vi "GUI_HamamatsuSpectrometer_v2.0.0.vi"() -> ()   [LabVIEW 2013]
uses:
  Shared/GUI_Template/GUI_master/tcp_new_data_event.ctl
  Shared/GUI_Template/GUI_master/tcp new data cluster.ctl
  <vilib>/Utility/miscctls.llb/LVOffsetAndMultiplierTypeDef.ctl
panel:
  out "wavelength::1":dbl[](array[numeric]) caption="wavelength"
  in  "Local Saving Path":path
  in  "stop":bool
  out "FWHM::1":dbl caption="FWHM" min=0.0 max=10000.0
  in  "BGlevel::1":dbl caption="BGlevel" min=0.0 max=10000.0
  out "MeanWavelength::1":dbl caption="MeanWavelength" min=0.0 max=10000.0
  out "lambda_r::1":dbl caption="lambda_r" min=0.0 max=10000.0
  out "lambda_b::1":dbl caption="lambda_b" min=0.0 max=10000.0
  out "lambda_width (SD)::1":dbl caption="lambda_width (SD)" min=0.0 max=10000.0
  out "AverageCountLevel::1":dbl caption="AverageCountLevel" min=0.0 max=10000.0
  in  "exposure::1":dbl caption="exposure" min=1.0 max=300.0
  in  "trigger::1":bool caption="trigger"
  in  "save::1":bool caption="save"
  in  "shotnumber":i32
  in  "Refresh Button":bool
  in  "GUIdevice 1":string="P2-AndorCam"
  out "counts::1":dbl[](array[numeric]) caption="counts"
  out "tcp data event":T1
  out "UDP error message":string caption="Device Errors"
  out "XY Graph":cluster{"Value":dbl[], "Value":dbl[]}[](graph)
  out "Intensity Graph":dbl[][](graph)
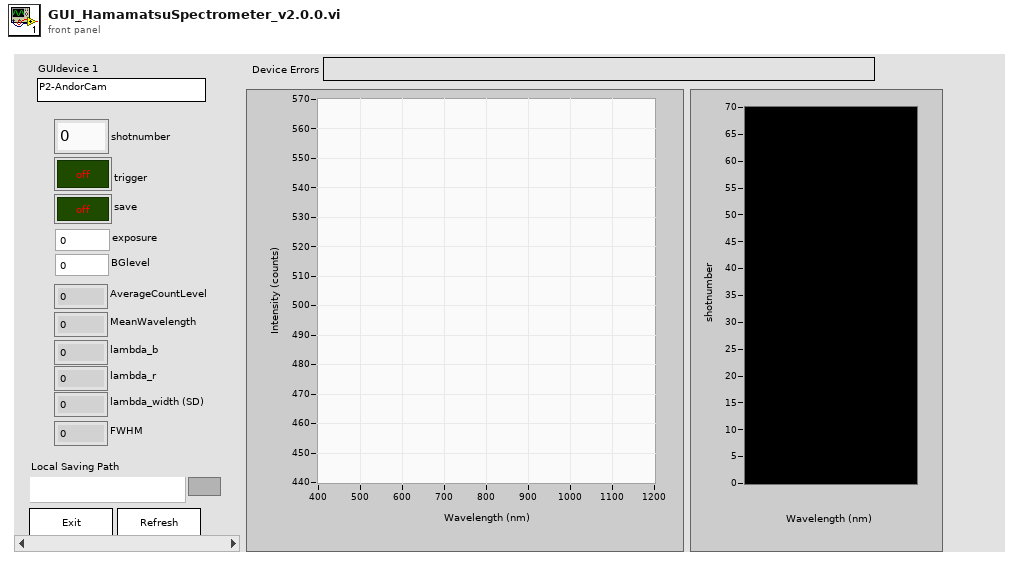
[diagram p1: front panel]
types:
  T1 = typedef "tcp_new_data_event.ctl" = refnum<user-event>
  T2 = enum32{"invalid app kind", "Development System", "Run Time System", "Student Edition", "Embedded LabVIEW", "Evaluation", "Custom"}
  T3 = typedef "tcp new data cluster.ctl" = cluster{"EventEnum":enum16{"new data", "connection status update"}, "Device name":string}
  T4 = enum32{"Invalid", "Standard", "Closed", "Hidden", "Minimized", "Maximized"}
  T5 = typedef "LVOffsetAndMultiplierTypeDef.ctl" = cluster{"Offset":dbl, "Multiplier":dbl}
  T6 = cluster{"Core":cluster{"Current VI Reference":refnum<vi>, "Close Panel on Exit?":bool}, "Your Boolean data":bool, "Your string data":string, "SuperGUI":cluster{"STOP queue":refnum<queue>, "SuperGUI ref":refnum<vi>}, "Graph":cluster{"XY Graph":cluster{"Value":dbl[], "Value":dbl[]}, "Intensity Graph":dbl[][], "Shot Number":i32}}
  T7 = cluster{"XY Graph":cluster{"Value":dbl[], "Value":dbl[]}, "Intensity Graph":dbl[][], "Shot Number":i32}
  T8 = cluster{"STOP queue":refnum<queue>, "SuperGUI ref":refnum<vi>}
  T9 = cluster{"Current VI Reference":refnum<vi>, "Close Panel on Exit?":bool}
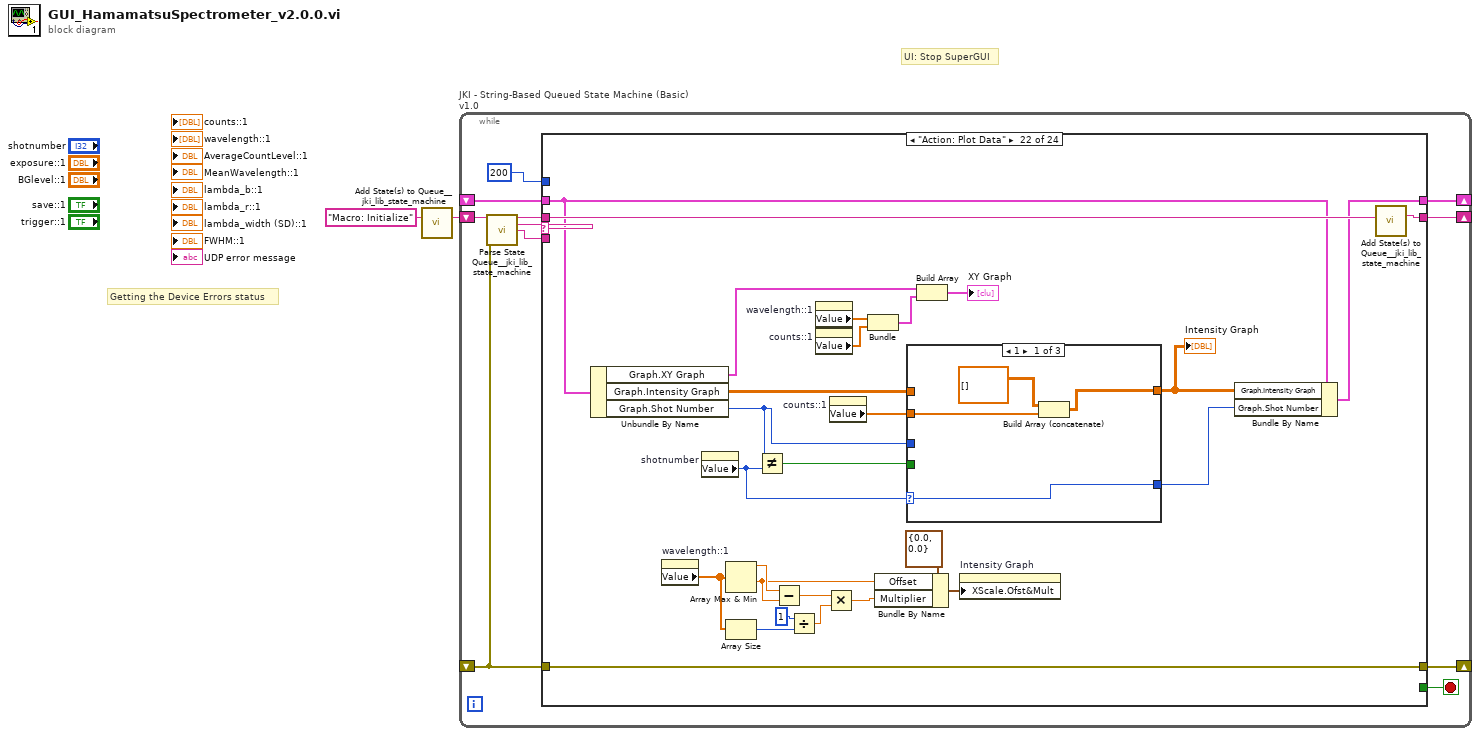
[diagram p0: block diagram]
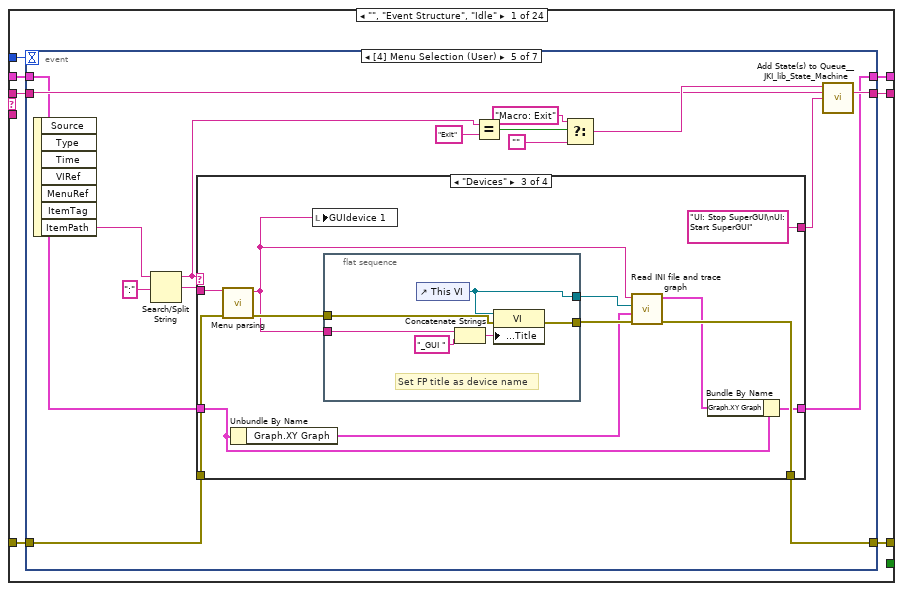
[diagram p2: hidden frame]
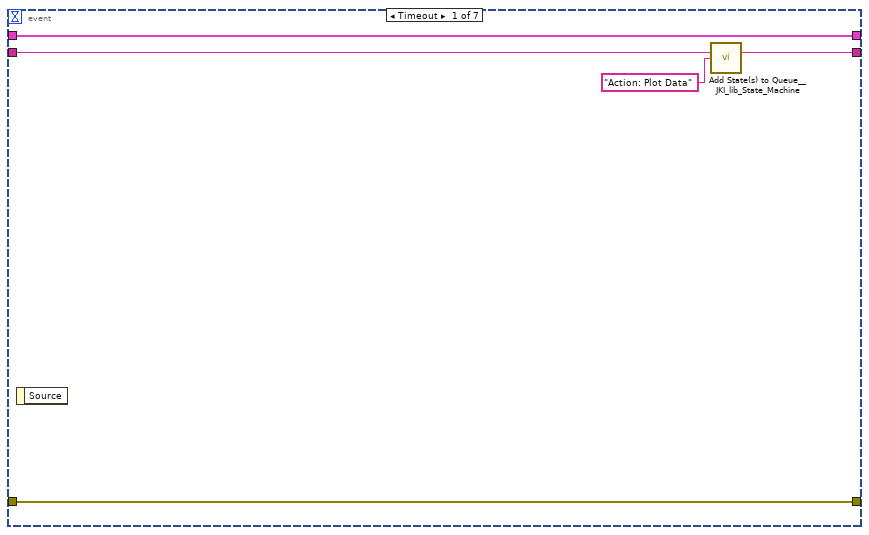
[diagram p3: hidden frame]
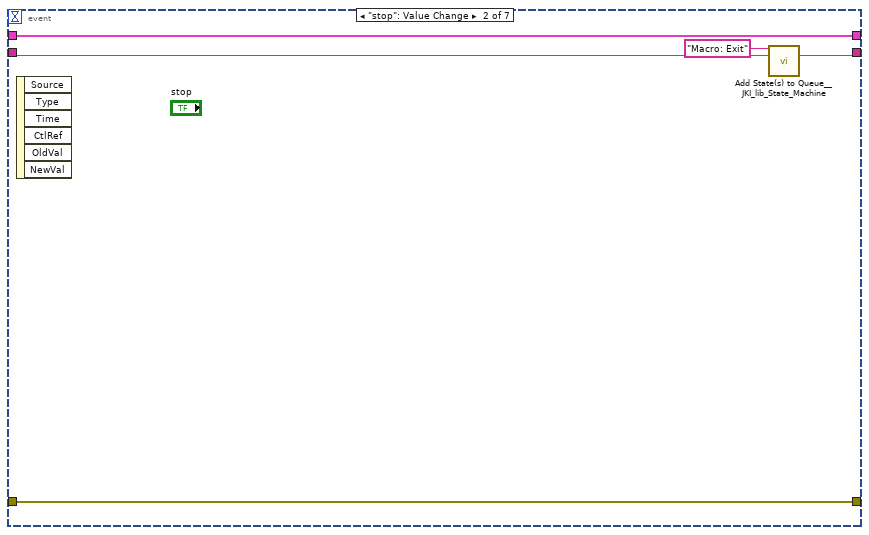
[diagram p4: hidden frame]
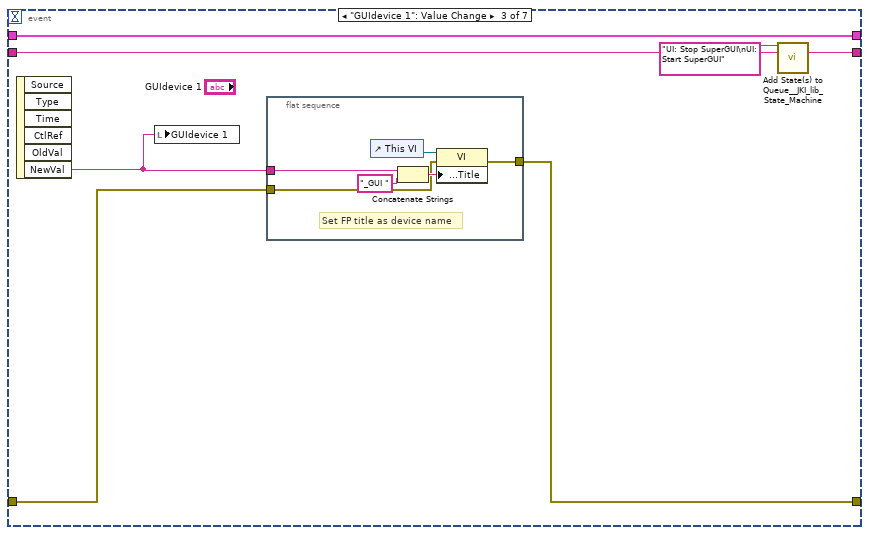
[diagram p5: hidden frame]
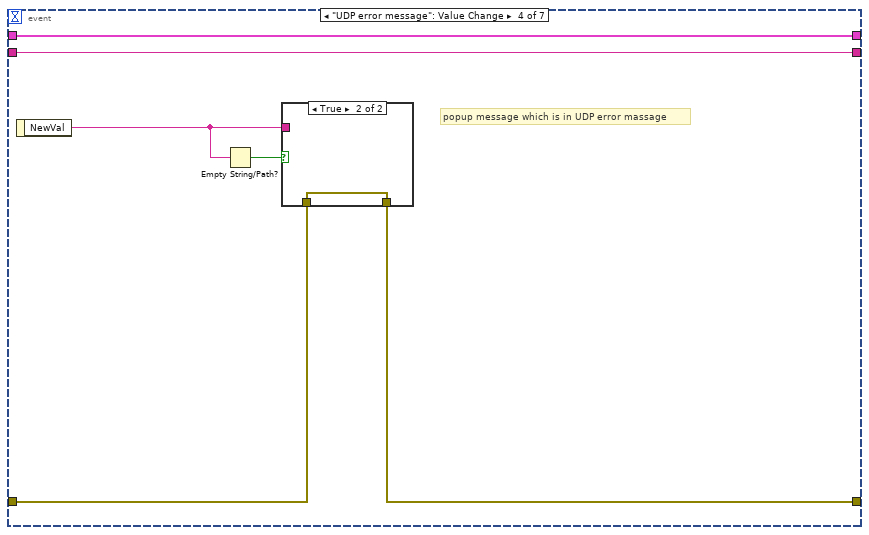
[diagram p6: hidden frame]
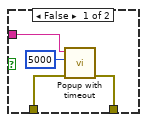
[diagram p7: hidden frame]
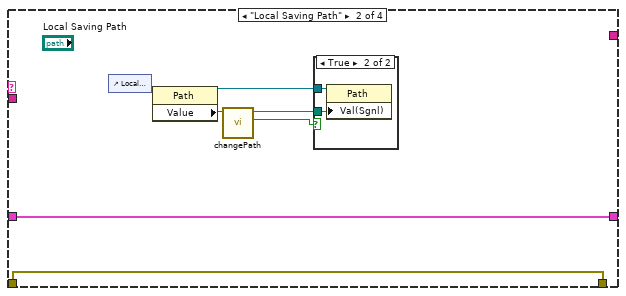
[diagram p9: hidden frame]
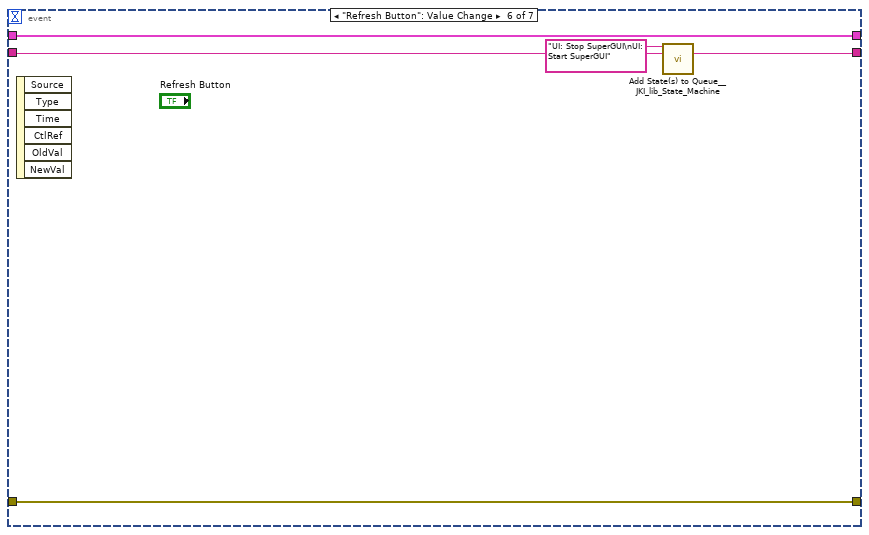
[diagram p12: hidden frame]
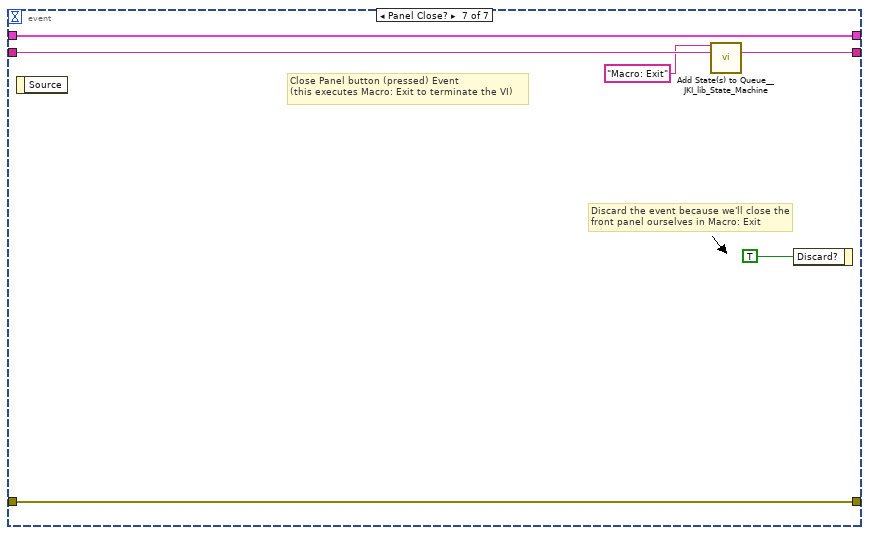
[diagram p13: hidden frame]
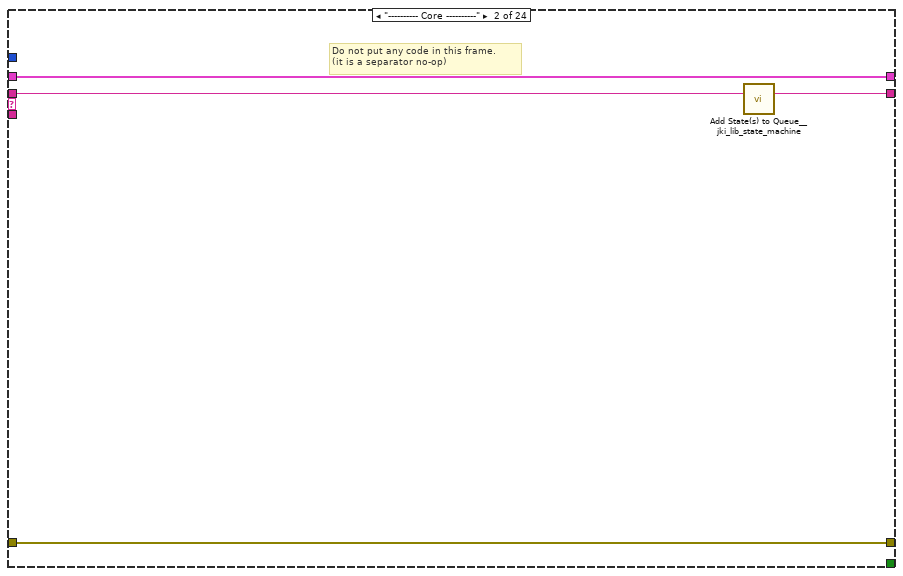
[diagram p14: hidden frame]
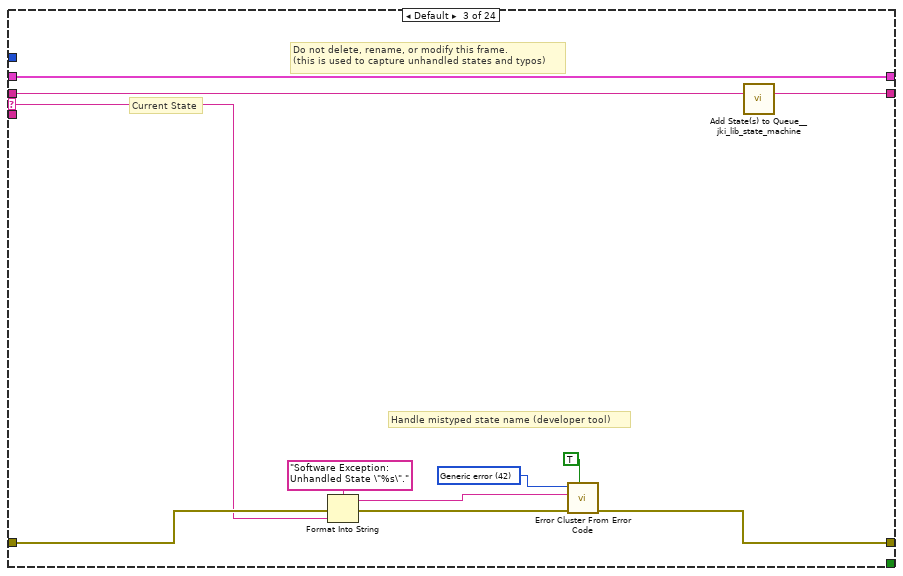
[diagram p15: hidden frame]
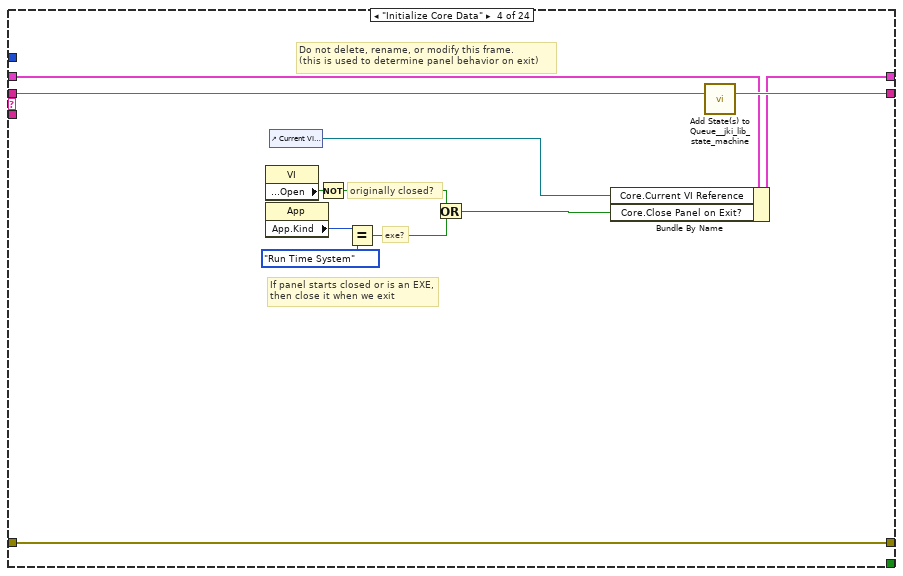
[diagram p16: hidden frame]
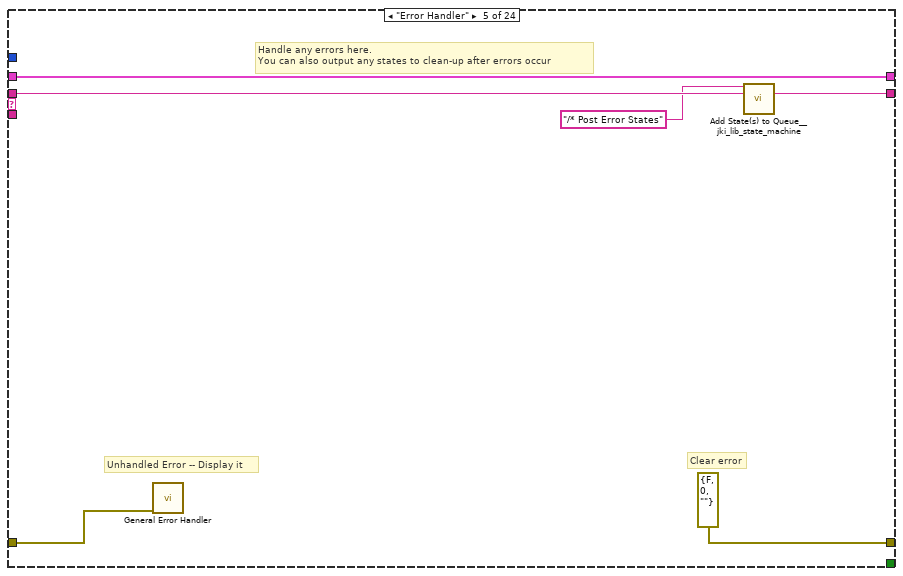
[diagram p17: hidden frame]
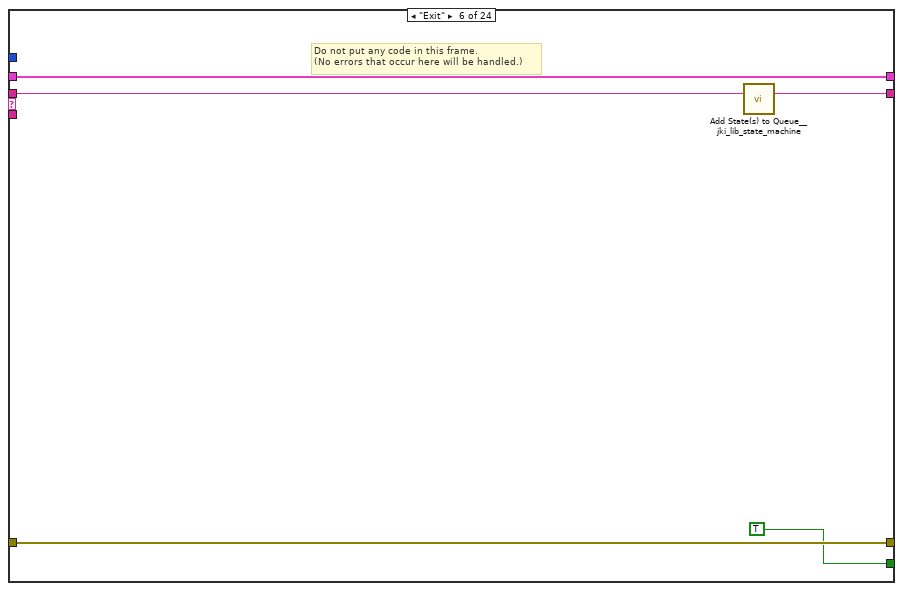
[diagram p18: hidden frame]
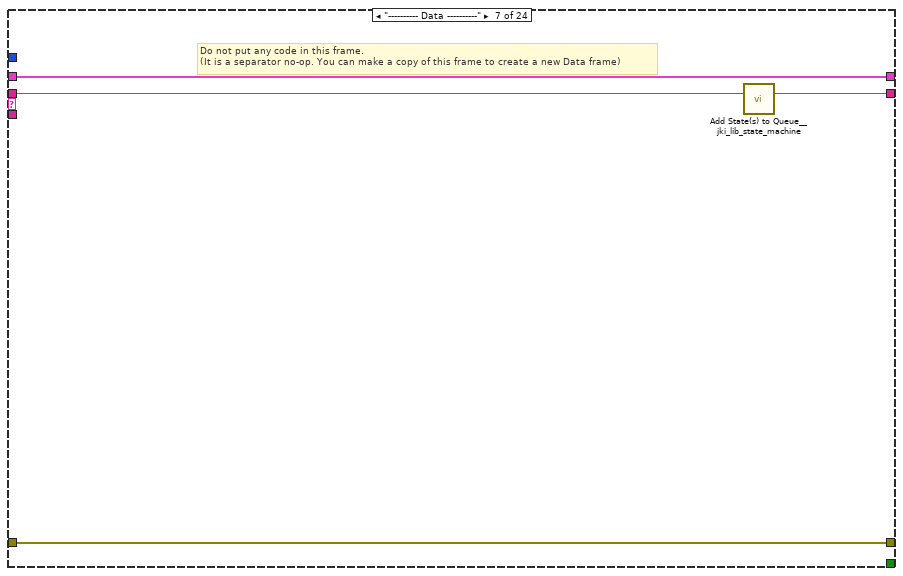
[diagram p19: hidden frame]
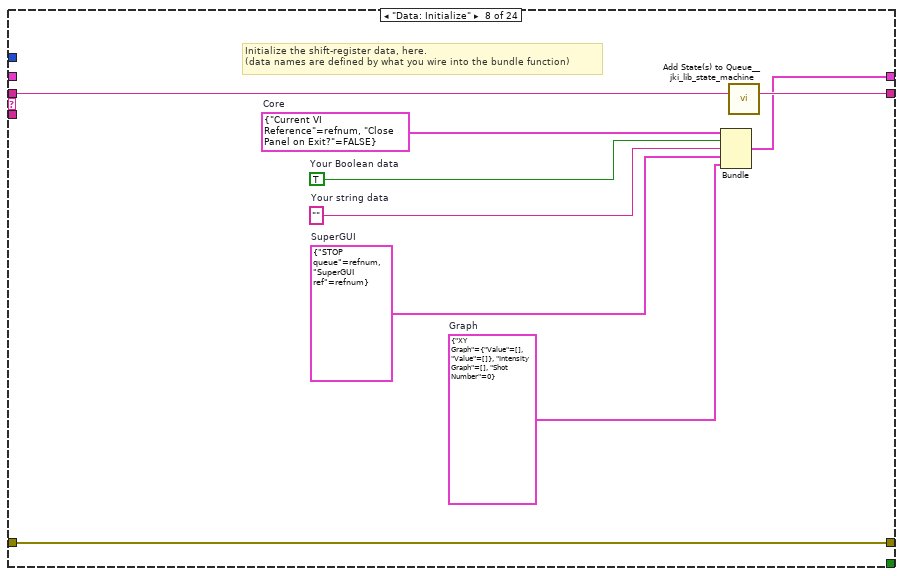
[diagram p20: hidden frame]
diagram:
  # "UI: Stop SuperGUI"
  # "Getting the Device Errors status"
  n1 = call <vilib>:"Add State(s) to Queue__jki_lib_state_machine.vi"("State(s) in (\"\")"="Macro: Initialize") -> ("States Out"=w2:string)  [unwired: 14 in]
  n2 = while "JKI - String-Based Queued State Machine (Basic) v1.0" {
    shift-right: [w6] -> _
    shift-left: _ -> [w5]
    shift-right: [w9] -> _
    shift-left: _ -> [w3]
    shift-right: [w8] -> _
    shift-left: w2 -> [w10]
    stop <- w7 stop-if-true
    n3 = call <vilib>:"Parse State Queue__jki_lib_state_machine.vi"("State Queue"=w10, "Error In (no error)"=w3) -> ("Remaining States"=w12:string, "Current State"=w13:string, "Arguments"=w11:string)  [unwired: 11 in]
    n4 = case shown="\"Action: Plot Data\"" w13 {
      selector: w13 -> [_ _ w116 _ _ _ _ _ _ _ _ _ _ _ _ _ _ _ _ _ _ _ _ _]
      tunnel: w12 -> [w20 w115 w120 w138 w144 w149 w153 w162 w168 w172 w176 w185 w221 w255 w263 w269 w280 w306 w311 w322 w326 w353 w376 w386]
      tunnel: w11 -> [_ _ _ _ _ _ _ _ _ _ _ _ _ _ _ w264 w274 _ _ _ _ _ _ _]
      tunnel: w5 -> [w18 w112 w118 w129 w141 w147 w150 _ w163 w169 w174 w183 w219 w246 w258 w267 w276 w303 w308 w319 w323 w345 w373 w380]
      tunnel: [w17 w113 w122 w135 errorcluster {"status"=FALSE, "code"=0, "source"=""} ("error out") w146 w151 w159 w164 w170 w173 w181 w216 w239 w256 w265 w277 w304 w309 w320 w324 w351 w374 w381] -> w9
      tunnel: w3 -> [w16 w113 w121 w135 w140 w146 w151 w159 w165 w170 w173 w182 w217 w240 w257 w266 w278 w304 w309 w320 w324 w351 w374 w382]
      tunnel: [w19 w114 w119 w137 w143 w148 w152 w161 w167 w171 w175 w184 w220 w254 w262 w268 w279 w305 w310 w321 w325 w352 w375 w385] -> w8
      tunnel: [_ _ _ _ _ TRUE _ _ _ _ _ _ _ _ _ _ _ _ _ _ _ _ _ _] -> w7
      tunnel: [w15 w112 w118 w136 w141 w147 w150 w160 w163 w169 w174 w183 w219 w245 w258 w267 w276 w303 w308 w319 w323 w344 w373 w379] -> w6
      tunnel: 200 ("time to wait (main loop)") -> [w14 _ _ _ _ _ _ _ _ _ _ _ _ _ _ _ _ _ _ _ _ _ _ _]
      frame "", "Event Structure", "Idle" {
        n5 = event shown="[4] Menu Selection (User)" {
          selector: _ -> [_ _ _ _ _ _ _]
          dyn-events: _ -> [_ _ _ _ _ _ _]
          timeout: w14 -> [_ _ _ _ _ _ _]
          tunnel: w20 -> [w25 w28 w34 w48 w65 w103 w111]
          tunnel: [w24 w27 w33 w48 w64 w102 w110] -> w19
          tunnel: w18 -> [w21 w30 w37 w49 w56 w105 w108]
          tunnel: [w22 w29 w35 w44 w58 w104 w109] -> w17
          tunnel: w16 -> [w22 w29 w36 w45 w59 w104 w109]
          tunnel: [w21 w30 w37 w49 w55 w105 w108] -> w15
          event Timeout {
            n6 = event-data() -> ()  [unwired: 1 in, 1 out]
            n7 = call <vilib>:"Add State(s) to Queue__JKI_lib_State_Machine.vi"("State(s) in (\"\")"=w25, "State(s) at Back (\"\")"="Action: Plot Data" ("State(s) in Front (\"\")")) -> ("States Out"=w24:string)  [unwired: 13 in]
          }
          event "stop": Value Change {
            n8 = event-data() -> ()  [unwired: 1 in, 6 out]
            n9 = call <vilib>:"Add State(s) to Queue__JKI_lib_State_Machine.vi"("State(s) in Front (\"\")"="Macro: Exit", "State(s) in (\"\")"=w28) -> ("States Out"=w27:string)  [unwired: 13 in]
          }
          event "GUIdevice 1": Value Change {
            n10 = event-data() -> ("NewVal"=w31:string)  [unwired: 1 in, 5 out]
            n11 = local write "GUIdevice 1"(w31) -> ()
            n12 = flat-sequence {
              tunnel: [w40] -> w35
              tunnel: w36 -> [w39]
              tunnel: w31 -> [w38]
              frame #0 {
                # "Set FP title as device name"
                n13 = control-ref of="This VI"() -> (w43:refnum<vi>)
                n14 = Concatenate Strings(w38, "_GUI ") -> (w42:string)
                n15 = property class="VI"(reference=w43, error in=w39, "Front Panel.Title"=w42) -> (error out=w40:errorcluster)  [unwired: 1 out]
              }
            }
            n16 = call <vilib>:"Add State(s) to Queue__JKI_lib_State_Machine.vi"("State(s) in Front (\"\")"="UI: Stop SuperGUI\nUI: Start SuperGUI", "State(s) in (\"\")"=w34) -> ("States Out"=w33:string)  [unwired: 13 in]
          }
          event "UDP error message": Value Change {
            # "popup message which is in UDP error massage"
            n17 = event-data() -> ("NewVal"=w46:string)  [unwired: 1 in]
            n18 = Empty String/Path?(string/path=w46) -> (empty?=w47:bool)
            n19 = case shown="True" w47 {
              tunnel: w46 -> [w53 _]
              tunnel: w45 -> [w52 w54]
              tunnel: [w51 w54] -> w44
              frame False {
                n20 = call "Popup with timeout.vi"("error"=w52, "timeout"=u32 5000, "message"=w53) -> ("error out"=w51:errorcluster)  [unwired: 8 in]
              }
              frame True {
              }
            }
          }
          event Menu Selection (User) {
            n21 = event-data() -> ("ItemPath"=w61:string)  [unwired: 1 in, 6 out]
            n22 = Search/Split String(string=w61, search string/char (-)=":") -> (substring before match=w57:string, match + rest of string=w60:string)  [unwired: 1 in, 1 out]
            n23 = case shown="\"Devices\"" w57 {
              tunnel: w60 -> [_ _ w92 _]
              tunnel: w59 -> [w72 w79 w91 w100]
              tunnel: [w72 w79 w86 w100] -> w58
              tunnel: [_ _ "UI: Stop SuperGUI\nUI: Start SuperGUI" _] -> w63
              tunnel: w56 -> [w71 w78 w84 w99]
              tunnel: [w71 w78 w82 w99] -> w55
              frame "", Default {
              }
              frame "Local Saving Path" {
                n24 = control-ref of="Local Saving Path"() -> (w77:refnum<vi>)
                n25 = property class="Path"(reference=w77) -> (reference out=w74:refnum<vi>, "Value"=w73:path)  [unwired: 1 in, 1 out]
                n26 = call "changePath.vi"("Local Saving in (h)"=w73) -> ("change (h)"=w75:bool, "Local Saving out (h)"=w76:path)  [unwired: 9 in]
                n27 = case shown="True" w75 {
                  tunnel: w74 -> [_ w81]
                  tunnel: w76 -> [_ w80]
                  frame False {
                  }
                  frame True {
                    n28 = property class="Path"(reference=w81, "Val(Sgnl)"=w80) -> ()  [unwired: 1 in, 2 out]
                  }
                }
              }
              frame "Devices" {
                n29 = call "Menu parsing.vi"("ItemPath 3"=w92) -> ("ItemPath 2"=w89:string)  [unwired: 9 in, 1 out]
                n30 = Unbundle By Name(w84) -> ("Graph.XY Graph"=w85:cluster{"Value":dbl[], "Value":dbl[]})
                n31 = local write "GUIdevice 1"(w89) -> ()
                n32 = flat-sequence {
                  tunnel: [w96] -> w87
                  tunnel: w91 -> [w95]
                  tunnel: w89 -> [w94]
                  tunnel: [w93] -> w88
                  frame #0 {
                    # "Set FP title as device name"
                    n33 = control-ref of="This VI"() -> (w93:refnum<vi>)
                    n34 = Concatenate Strings(w94, "_GUI ") -> (w98:string)
                    n35 = property class="VI"(reference=w93, error in=w95, "Front Panel.Title"=w98) -> (error out=w96:errorcluster)  [unwired: 1 out]
                  }
                }
                n36 = call "Read INI file and trace graph.vi"("error in (no error)"=w87, "XY Graph in"=w85, "This VI"=w88, "Device Name"=w89) -> ("error out"=w86:errorcluster, "XY Graph out"=w83:cluster{"Value":dbl[], "Value":dbl[]})  [unwired: 6 in]
                n37 = Bundle By Name(cluster=w84, "Graph.XY Graph"=w83) -> (w82:T6)
              }
              frame "Exit" {
              }
            }
            n38 = Equal?(x=w57, y="Exit") -> (x = y?=w69:bool)
            n39 = Select(t="Macro: Exit", s=w69, f="") -> (s? t:f=w66:string)
            n40 = call <vilib>:"Add State(s) to Queue__JKI_lib_State_Machine.vi"("State(s) in Front (\"\")"=w66, "State(s) in (\"\")"=w65, "State(s) at Back (\"\")"=w63) -> ("States Out"=w64:string)  [unwired: 12 in]
          }
          event "Refresh Button": Value Change {
            n41 = event-data() -> ()  [unwired: 1 in, 6 out]
            n42 = call <vilib>:"Add State(s) to Queue__JKI_lib_State_Machine.vi"("State(s) in Front (\"\")"="UI: Stop SuperGUI\nUI: Start SuperGUI", "State(s) in (\"\")"=w103) -> ("States Out"=w102:string)  [unwired: 13 in]
          }
          event Panel Close? {
            # "Discard the event because we'll close the front panel ourselves in Macro: Exit"
            # "Close Panel button (pressed) Event\n(this executes Macro: Exit to terminate the VI)"
            n43 = event-data() -> ()  [unwired: 1 in, 1 out]
            n44 = call <vilib>:"Add State(s) to Queue__JKI_lib_State_Machine.vi"("State(s) in Front (\"\")"="Macro: Exit", "State(s) in (\"\")"=w111) -> ("States Out"=w110:string)  [unwired: 13 in]
            n45 = event-data("Discard?"=TRUE) -> ()  [unwired: 1 in, 1 out]
          }
        }
      }
      frame "---------- Core ----------" {
        # "Do not put any code in this frame.\n(it is a separator no-op)"
        n46 = call <vilib>:"Add State(s) to Queue__jki_lib_state_machine.vi"("State(s) in (\"\")"=w115) -> ("States Out"=w114:string)  [unwired: 14 in]
      }
      frame Default {
        w125 = 42 items=["No error", "Argument error", "Memory is full", "Out of zone", "End of file", "File already open", "Generic file I/O error", "File not found", "File permission error", "Disk is full", "Duplicate path", "Too many files open", "System feature not enabled", "Resource file not found", "Cannot add resource", "Resource not found", "Image not found", "Image memory error", "Pen does not exist", "Config type invalid", "Config token not found", "Config parse error", "Config memory error", "Bad external code format", "Bad external code offset", "External code not present", "Null window", "Destroy window error", "Null menu", "Print aborted", "Bad print record", "Print driver error", "Windows error during printing", "Memory error during printing", "Print dialog error", "Generic print error", "Invalid device refnum", "Device not found", "Device parameter error", "Device unit error", "Cannot open device", "Device call aborted", "Generic error", "Cancelled by user", "Object ID too low", "Object ID too high", "Object not in heap", "Unknown heap", "Unknown object (invalid DefProc)", "Unknown object (DefProc not in table)", "Message out of range", "Invalid (null) method", "Unknown message", "Manager call not supported", "Bad address", "Network operation in progress", "Network operation timed out", "Connection is busy", "Network attribute not supported", "Network error", "Address in use", "System out of memory", "Connection aborted", "Connection refused", "Not connected", "Already connected", "Connection closed", "Initialization error (interapplication manager)", "Bad occurrence", "Wait on unbound occurrence handler", "Occurrence queue overflow", "Datalog type conflict", "Unused", "Unrecognized type (interapplication manager)", "Memory corrupt", "Failed to make temporary DLL", "Old CIN version", "Drag socket not found", "Failed to load drop-object", "Failed to register OLE object", "Failed to release OLE object", "Format specifier type mismatch", "Unknown format specifier", "Too few format specifiers", "Too many format specifiers", "Scan failed", "Newer CIN version", "Error converting to variant", "Runtime menu error", "Password tampered", "Variant attribute not found", "Incompatible variant data type", "Event data is not available", "Event Store is not present", "Occurrence is not found", "Event Queue is not created", "Event info is not available", "Refnum passed is NULL", "Error retrieving Class GUID", "Error retrieving CoClass GUID", "Error retrieving TypeLib GUID.", "Bad built application magic bytes.", "Specific driver is different from the specific driver associated with the Logical Name.", "There is no session opened to the class driver.", "Max Error", "MAX - Error with config objects", "MAX - Error loading configuration", "MAX - Group not supported"]
        # "Current State"
        # "Do not delete, rename, or modify this frame.\n(this is used to capture unhandled states and typos)"
        # "Handle mistyped state name (developer tool)"
        n47 = Format Into String(format string="Software Exception: Unhandled State \"%s\"." ("message"), error in=w121, w116) -> (resulting string=w124:string, error out=w123:errorcluster)  [unwired: 1 in]
        n48 = call <vilib>:"Error Cluster From Error Code.vi"("show call chain? (False)"=TRUE, "error in (no error)"=w123, "error message (\"\")"=w124, "error code (0)"=w125) -> ("error out"=w122:errorcluster)  [unwired: 5 in]
        n49 = call <vilib>:"Add State(s) to Queue__jki_lib_state_machine.vi"("State(s) in (\"\")"=w120) -> ("States Out"=w119:string)  [unwired: 14 in]
      }
      frame "Initialize Core Data" {
        # "Do not delete, rename, or modify this frame.\n(this is used to determine panel behavior on exit)"
        # "originally closed?"
        # "exe?"
        # "If panel starts closed or is an EXE, then close it when we exit"
        n50 = property class="VI"() -> ("Front Panel.Open"=w134:bool)  [unwired: 2 in, 2 out]
        n51 = property class="App"() -> ("App.Kind"=w133:T2)  [unwired: 2 in, 2 out]
        n52 = control-ref of="Current VI Reference"() -> (w127:refnum<vi>)
        n53 = Not(x=w134) -> (.not. x?=w131:bool)
        n54 = Equal?(x=w133, y=T2."Run Time System" ("Application:Kind")) -> (x = y?=w130:bool)
        n55 = Or(x=w131, y=w130) -> (x .or. y?=w128:bool)
        n56 = Bundle By Name(cluster=w129, "Core.Current VI Reference"=w127, "Core.Close Panel on Exit?"=w128) -> (w136:T6)
        n57 = call <vilib>:"Add State(s) to Queue__jki_lib_state_machine.vi"("State(s) in (\"\")"=w138) -> ("States Out"=w137:string)  [unwired: 14 in]
      }
      frame "Error Handler" {
        # "Unhandled Error -- Display it"
        # "Handle any errors here.\nYou can also output any states to clean-up after errors occur"
        # "Clear error"
        n58 = call <vilib>:"General Error Handler.vi"("error in (no error)"=w140) -> ()  [unwired: 10 in, 5 out]
        n59 = call <vilib>:"Add State(s) to Queue__jki_lib_state_machine.vi"("State(s) in Front (\"\")"="/* Post Error States", "State(s) in (\"\")"=w144) -> ("States Out"=w143:string)  [unwired: 13 in]
      }
      frame "Exit" {
        # "Do not put any code in this frame.\n(No errors that occur here will be handled.)"
        n60 = call <vilib>:"Add State(s) to Queue__jki_lib_state_machine.vi"("State(s) in (\"\")"=w149) -> ("States Out"=w148:string)  [unwired: 14 in]
      }
      frame "---------- Data ----------" {
        # "Do not put any code in this frame.\n(It is a separator no-op. You can make a copy of this frame to create a new Data frame)"
        n61 = call <vilib>:"Add State(s) to Queue__jki_lib_state_machine.vi"("State(s) in (\"\")"=w153) -> ("States Out"=w152:string)  [unwired: 14 in]
      }
      frame "Data: Initialize" {
        w154 = T7 {"XY Graph"={"Value"=[], "Value"=[]}, "Intensity Graph"=[], "Shot Number"=0}  # Graph
        w155 = T8 {"STOP queue"=refnum, "SuperGUI ref"=refnum}  # SuperGUI
        w156 = T9 {"Current VI Reference"=refnum, "Close Panel on Exit?"=FALSE}  # Core
        w158 = TRUE  # Your Boolean data
        w157 = ""  # Your string data
        # "Initialize the shift-register data, here.\n(data names are defined by what you wire into the bundle function)"
        n62 = Bundle("Core"=w156, "Your Boolean data"=w158, "Your string data"=w157, "SuperGUI"=w155, "Graph"=w154) -> (w160:T6)  [unwired: 1 in]
        n63 = call <vilib>:"Add State(s) to Queue__jki_lib_state_machine.vi"("State(s) in (\"\")"=w162) -> ("States Out"=w161:string)  [unwired: 14 in]
      }
      frame "Data: Cleanup" {
        # "Cleanup any data and references, here.\n(this is called automatically, by the Macro: Exit)"
        n64 = Unbundle By Name(w163) -> ("Core.Current VI Reference"=w166:refnum<vi>)
        n65 = Close Reference(reference=w166, error in (no error)=w165) -> (error out=w164:errorcluster)
        n66 = call <vilib>:"Add State(s) to Queue__jki_lib_state_machine.vi"("State(s) in (\"\")"=w168) -> ("States Out"=w167:string)  [unwired: 14 in]
      }
      frame "---------- UI ----------" {
        # "Do not put any code in this frame.\n(It is a separator no-op. You can make a copy of this frame to create a new UI frame)"
        n67 = call <vilib>:"Add State(s) to Queue__jki_lib_state_machine.vi"("State(s) in (\"\")"=w172) -> ("States Out"=w171:string)  [unwired: 14 in]
      }
      frame "UI: Initialize" {
        # "Initialize the User Interface, here.\n(this is called automatically, by the Macro: Init)"
        n68 = call <vilib>:"Add State(s) to Queue__jki_lib_state_machine.vi"("State(s) in (\"\")"=w176) -> ("States Out"=w175:string)  [unwired: 14 in]
      }
      frame "UI: Update Device List" {
        # "menu is not set visible in vi properties"
        n69 = for {
          shift-right: [w187] -> w177
          shift-left: string[] [] -> [w188]
          tunnel: string[] ["HamamatsuSpectrometer", "HamamatsuSpectrometerXP", "OceanOpticsSpectrometer", "HamamatsuSpectrometerDAQ", "Thorlabs CCS175 Spectrometer", "Qred", "StellarNet Black-Comet"] -> [w186] mode=indexing
          n70 = call "getDevices.vi"("Device Class"=w186) -> ("All Devices"=w189:string[])
          n71 = Build Array (concatenate)(w188, w189) -> (w187:string[])
        }
        n72 = Empty Array?(array=w177) -> (empty?=w180:bool)
        n73 = case shown="False" w180 {
          tunnel: w182 -> [w192 w215]
          tunnel: [w191 w215] -> w181
          tunnel: w177 -> [w190 _]
          frame False {
            n74 = Current VI's Menubar() -> (w195:refnum<k9>)
            n75 = Get Menu Item Info(7:"Devices" ("item tag"), 8:w192, 11:w195) -> (0:w201:errorcluster, 3:w197:refnum<k9>)  [unwired: 5 out]
            n76 = Set Menu Item Info(7:"Devices" ("item tag"), 8:w201, 9:TRUE ("enabled"), 11:w197) -> (0:w200:errorcluster, 3:w199:refnum<k9>)  [unwired: 3 in]
            n77 = First Call?() -> (First Call?: T/F=w193:bool)
            n78 = case shown="True" w193 {
              tunnel: w199 -> [_ w207]
              tunnel: w190 -> [_ w206]
              tunnel: w200 -> [w202 w204]
              tunnel: [w202 w203] -> w191
              frame False {
              }
              frame True {
                n79 = for {
                  tunnel: [w214] -> w208
                  tunnel: w206 -> [w212] mode=indexing
                  tunnel: w207 -> [w211]
                  tunnel: [w210] -> w205
                  tunnel: w204 -> [w209]
                  n80 = Insert Menu Items(5:"Devices" ("menu tag"), 6:w209, 7:w212, 8:w212, 9:w211) -> (0:w210:errorcluster, 3:w214:refnum<k9>)  [unwired: 1 in, 1 out]
                }
                n81 = Enable Menu Tracking(2:w205, 4:w208) -> (0:w203:errorcluster)  [unwired: 1 in, 1 out]
              }
            }
          }
          frame True {
          }
        }
        n82 = call <vilib>:"Add State(s) to Queue__jki_lib_state_machine.vi"("State(s) in (\"\")"=w185) -> ("States Out"=w184:string)  [unwired: 14 in]
      }
      frame "UI: Get Device Name" {
        n83 = First Call?() -> (First Call?: T/F=w218:bool)
        n84 = case shown="True" w218 {
          tunnel: w217 -> [w222 w224]
          tunnel: [w222 w223] -> w216
          frame False {
          }
          frame True {
            n85 = disable-structure "Get Device name from control for vi mode\nand command line arg for exe" shown="RUN_TIME_ENGINE==True" {
              disable-tunnel: w224 -> [_ w226]
              disable-tunnel: [_ w225] -> w223
              frame condition #0 (active) {
              }
              frame condition #1 {
                n86 = control-ref of="This Application"() -> (w234:refnum<vi>)
                n87 = property class="App"(reference=w234) -> ("App.Args"=w233:string[])  [unwired: 1 in, 2 out]
                n88 = Index Array(array=w233, index #1=1 ("index")) -> (element #1=w227:string)  [unwired: 2 in, 2 out]
                n89 = Empty String/Path?(string/path=w227) -> (empty?=w231:bool)
                n90 = control-ref of="This VI"() -> (w230:refnum<vi>)
                n91 = case shown="False" w231 {
                  tunnel: w227 -> [w235 _]
                  frame False {
                    n92 = local write "GUIdevice 1"(w235) -> ()
                  }
                  frame True {
                  }
                }
                n93 = Concatenate Strings(w227, "_GUI ") -> (w229:string)
                n94 = property class="VI"(reference=w230, error in=w226, "Front Panel.Title"=w229) -> (error out=w225:errorcluster)  [unwired: 1 out]
              }
            }
          }
        }
        n95 = call <vilib>:"Add State(s) to Queue__jki_lib_state_machine.vi"("State(s) in (\"\")"=w221) -> ("States Out"=w220:string)  [unwired: 14 in]
      }
      frame "UI: Start SuperGUI" {
        # "create stop queue for supergui and its clones"
        # "x100 abort will be dependent on caller VI\nx80 abort will be independent of caller vi, this will abort vi when labview is closed."
        # "Start SuperGUI asynchronous way"
        n96 = vi-ref "GUI_Master_subvi_reentrant_queues.vi"() -> (w238:refnum<vi>)
        n97 = property class="VI"(reference=w238) -> ("Path"=w237:path)  [unwired: 1 in, 2 out]
        n98 = Create User Event(user event datatype=T3 {"EventEnum"=enum."new data", "Device name"="Device name"} ("New Event"), error in=w240) -> (user event=w241:refnum<user-event>, error out=w247:errorcluster)
        "tcp data event" <- w241
        n99 = control-ref of="This Application"() -> (w244:refnum<vi>)
        n100 = control-ref of="This VI"() -> (w243:refnum<vi>)
        n101 = Open VI Reference(type specifier VI Refnum (for type only)=refnum<vi> refnum, vi path=w237, options=256) -> (vi reference=w253:refnum<vi>, error out=w252:errorcluster)  [unwired: 3 in]
        n102 = register-events(w241) -> ()  [unwired: 2 in, 2 out]
        n103 = call "supergui create stop queue.vi"() -> ("STOP Queue out"=w249:refnum<queue>)  [unwired: 11 in]
        n104 = Current VI's Menubar() -> (w242:refnum<k9>)
        n105 = call-by-ref "Start Asynchronous Call"(reference=w253, error in=w252, "STOP Queue in"=w249, "This Application"=w244, 8:"error in (no error)"=w247, "tcp data event"=w241, "Caller menu reference"=w242, "Caller VI ref"=w243) -> (reference out=w236:refnum<vi>, error out=w239:errorcluster)  [unwired: 5 in, 1 out]
        n106 = Bundle By Name(cluster=w246, "SuperGUI.SuperGUI ref"=w236, "SuperGUI.STOP queue"=w249) -> (w245:T6)
        n107 = call <vilib>:"Add State(s) to Queue__jki_lib_state_machine.vi"("State(s) in (\"\")"=w255) -> ("States Out"=w254:string)  [unwired: 14 in]
      }
      frame "UI: Stop SuperGUI" {
        # "Stop Supergui Clone and wait until it exit properly"
        n108 = Unbundle By Name(w258) -> ("SuperGUI.SuperGUI ref"=w260:refnum<vi>, "SuperGUI.STOP queue"=w259:refnum<queue>)
        n109 = Release Queue(queue=w259, error in (no error)=w257) -> (error out=w261:errorcluster)  [unwired: 1 in, 2 out]
        n110 = call-by-ref "Wait On Asynchronous Call"(reference=w260, error in=w261) -> ("error out"=w256:errorcluster)  [unwired: 11 in, 2 out]
        n111 = call <vilib>:"Add State(s) to Queue__jki_lib_state_machine.vi"("State(s) in (\"\")"=w263) -> ("States Out"=w262:string)  [unwired: 14 in]
      }
      frame "UI: Cursor Set" {
        # "Argument"
        # "Set and Unset Cursor Busy.\n(Usage: \"UI: Cursor Set >> Busy|Idle\")"
        n112 = case shown="\"Idle\", Default" w264 {
          tunnel: w266 -> [w271 w273]
          tunnel: [w270 w272] -> w265
          frame "Idle", Default {
            n113 = call <vilib>:"Unset Busy.vi"("error in (no error)"=w271) -> ("error out"=w270:errorcluster)  [unwired: 10 in]
          }
          frame "Busy" {
            n114 = call <vilib>:"Set Busy.vi"("error in (no error)"=w273) -> ("error out"=w272:errorcluster)  [unwired: 9 in, 1 out]
          }
        }
        n115 = call <vilib>:"Add State(s) to Queue__jki_lib_state_machine.vi"("State(s) in (\"\")"=w269) -> ("States Out"=w268:string)  [unwired: 14 in]
      }
      frame "UI: Front Panel State" {
        # "Argument"
        # "Set Front Panel Open or Closed\n(Usage: \"UI: Front Panel State >> Open|Close\")"
        n116 = Unbundle By Name(w276) -> ("Core.Current VI Reference"=w275:refnum<vi>)
        n117 = case shown="\"Close\"" w274 {
          tunnel: w278 -> [w284 w297]
          tunnel: [w286 w298] -> w277
          tunnel: w275 -> [w285 w295]
          frame "Open", Default {
            n118 = property class="VI"(reference=w285, error in=w284) -> (reference out=w282:refnum<vi>, error out=w283:errorcluster, "Front Panel.Open"=w281:bool)
            n119 = case shown="False" w281 {
              tunnel: [w289 w292] -> w286
              tunnel: w283 -> [w288 w292]
              tunnel: w282 -> [w287 _]
              frame False {
                n120 = invoke class="VI" method="FP.Open"(reference=w287, error in=w288, "Activate"=TRUE, "State"=T4."Standard") -> (error out=w289:errorcluster)  [unwired: 1 in, 4 out]
              }
              frame True {
              }
            }
          }
          frame "Close" {
            n121 = property class="VI"(reference=w295, error in=w297) -> (reference out=w294:refnum<vi>, error out=w296:errorcluster, "Front Panel.Open"=w293:bool)
            n122 = case shown="True" w293 {
              tunnel: [w299 w302] -> w298
              tunnel: w296 -> [w299 w301]
              tunnel: w294 -> [_ w300]
              frame False {
              }
              frame True {
                n123 = invoke class="VI" method="FP.Close"(reference=w300, error in=w301) -> (error out=w302:errorcluster)  [unwired: 1 in, 2 out]
              }
            }
          }
        }
        n124 = call <vilib>:"Add State(s) to Queue__jki_lib_state_machine.vi"("State(s) in (\"\")"=w280) -> ("States Out"=w279:string)  [unwired: 14 in]
      }
      frame "---------- Macro ----------" {
        # "Do not put any code in this frame.\n(It is a separator no-op. You can make a copy of this frame to create a new Macro frame)"
        n125 = call <vilib>:"Add State(s) to Queue__jki_lib_state_machine.vi"("State(s) in (\"\")"=w306) -> ("States Out"=w305:string)  [unwired: 14 in]
      }
      frame "Macro: Initialize" {
        # "Initialization Macro\n(This is called once, when the VI starts)"
        n126 = call <vilib>:"Add State(s) to Queue__jki_lib_state_machine.vi"("State(s) in Front (\"\")"="Data: Initialize\nInitialize Core Data\nUI: Initialize\nUI: Update Device List\nUI: Get Device Name\nUI: Start SuperGUI\nUI: Front Panel State >> Open\nAction: Load Reference Trace", "State(s) in (\"\")"=w311) -> ("States Out"=w310:string)  [unwired: 13 in]
      }
      frame "Macro: Exit" {
        # "Exit Macro\n(This is called once, when the VI exits)"
        n127 = Unbundle By Name(w319) -> ("Core.Close Panel on Exit?"=w318:bool)
        n128 = Select(t="UI: Front Panel State >> Close", s=w318, f="") -> (s? t:f=w315:string)
        n129 = call <vilib>:"Add State(s) to Queue__jki_lib_state_machine.vi"("State(s) in Front (\"\")"="UI: Stop SuperGUI" ("State(s) in Front (\"\")"), "State(s) in (\"\")"=w315, "State(s) at Back (\"\")"="Data: Cleanup\nExit") -> ("States Out"=w313:string)  [unwired: 12 in]
        n130 = call <vilib>:"Add State(s) to Queue__jki_lib_state_machine.vi"("State(s) in Front (\"\")"=w313, "State(s) in (\"\")"=w322) -> ("States Out"=w321:string)  [unwired: 13 in]
      }
      frame "---------- Action ----------" {
        # "Template Separator\n(You can make a copy of, or modify, this frame)"
        n131 = call <vilib>:"Add State(s) to Queue__jki_lib_state_machine.vi"("State(s) in (\"\")"=w326) -> ("States Out"=w325:string)  [unwired: 14 in]
      }
      frame "Action: Plot Data" {
        n132 = Unbundle By Name(w345) -> ("Graph.XY Graph"=w342:cluster{"Value":dbl[], "Value":dbl[]}, "Graph.Intensity Graph"=w350:dbl[][], "Graph.Shot Number"=w348:i32)
        n133 = property on="wavelength::1" class="Arr (strict)"() -> ("Value"=w327:dbl[])  [unwired: 2 in, 2 out]
        n134 = property on="shotnumber" class="DigNum (strict)"() -> ("Value"=w346:i32)  [unwired: 2 in, 2 out]
        n135 = Array Max & Min(array=w327) -> (max value=w334:dbl, min value=w329:dbl)  [unwired: 2 out]
        n136 = Array Size(array=w327) -> (size(s)=w336:i32)
        n137 = Not Equal?(x=w348, y=w346) -> (x != y?=w347:bool)
        n138 = Subtract(x=w334, y=w329) -> (x-y=w333:dbl)
        n139 = Divide(x=1, y=w336) -> (x/y=w332:dbl)
        n140 = property on="wavelength::1" class="Arr (strict)"() -> ("Value"=w341:dbl[])  [unwired: 2 in, 2 out]
        n141 = property on="counts::1" class="Arr (strict)"() -> ("Value"=w340:dbl[])  [unwired: 2 in, 2 out]
        n142 = Multiply(x=w333, y=w332) -> (x*y=w328:dbl)
        n143 = property on="counts::1" class="Arr (strict)"() -> ("Value"=w349:dbl[])  [unwired: 2 in, 2 out]
        n144 = Bundle("Value"=w341, "Value"=w340) -> (w339:cluster{"Value":dbl[], "Value":dbl[]})  [unwired: 1 in]
        n145 = Bundle By Name(cluster=T5 {"Offset"=0.0, "Multiplier"=0.0} ("X Scale.Offset and Multiplier"), "Offset"=w329, "Multiplier"=w328) -> (w330:T5)
        n146 = case shown="1" w346 {
          selector: w346 -> [w354 w358 w362]
          tunnel: w350 -> [_ w359 w366]
          tunnel: w349 -> [w356 _ w365]
          tunnel: [w355 w359 w364] -> w337
          tunnel: w347 -> [_ _ w363]
          tunnel: [w354 w358 w361] -> w343
          tunnel: w348 -> [_ _ w360]
          frame 1 {
            n147 = Build Array (concatenate)(dbl[][] [] ("wavelength 2"), w356) -> (w355:dbl[][])
          }
          frame 0 {
          }
          frame 2, Default {
            n148 = case shown="True" w363 {
              tunnel: w366 -> [w368 w372]
              tunnel: [w368 w371] -> w364
              tunnel: w365 -> [_ w370]
              tunnel: w362 -> [_ w369]
              tunnel: [w367 w369] -> w361
              tunnel: w360 -> [w367 _]
              frame False {
              }
              frame True {
                n149 = Build Array (concatenate)(w372, w370) -> (w371:dbl[][])
              }
            }
          }
        }
        "Intensity Graph" <- w337
        n150 = Build Array(w342, w339) -> (→"XY Graph":cluster{"Value":dbl[], "Value":dbl[]}[])
        n151 = property on="Intensity Graph" class="IntGraph (strict)"("XScale.Ofst&Mult"=w330) -> ()  [unwired: 2 in, 2 out]
        n152 = Bundle By Name(cluster=w345, "Graph.Intensity Graph"=w337, "Graph.Shot Number"=w343) -> (w344:T6)
        n153 = call <vilib>:"Add State(s) to Queue__jki_lib_state_machine.vi"("State(s) in (\"\")"=w353) -> ("States Out"=w352:string)  [unwired: 14 in]
      }
      frame "New Category: 2" {
        # "Your code here.\n(You can make a copy of, or modify, this frame)"
        n154 = call <vilib>:"Add State(s) to Queue__jki_lib_state_machine.vi"("State(s) in (\"\")"=w376) -> ("States Out"=w375:string)  [unwired: 14 in]
      }
      frame "Action: Load Reference Trace" {
        # "Your code here.\n(You can make a copy of, or modify, this frame)"
        n155 = Unbundle By Name(w380) -> ("Graph.XY Graph"=w384:cluster{"Value":dbl[], "Value":dbl[]})
        n156 = local read "GUIdevice 1"() -> (w377:string)
        n157 = control-ref of="This VI"() -> (w378:refnum<vi>)
        n158 = call "Read INI file and trace graph.vi"("error in (no error)"=w382, "XY Graph in"=w384, "This VI"=w378, "Device Name"=w377) -> ("error out"=w381:errorcluster, "XY Graph out"=w383:cluster{"Value":dbl[], "Value":dbl[]})  [unwired: 6 in]
        n159 = call <vilib>:"Add State(s) to Queue__jki_lib_state_machine.vi"("State(s) in (\"\")"=w386) -> ("States Out"=w385:string)  [unwired: 14 in]
        n160 = Bundle By Name(cluster=w380, "Graph.XY Graph"=w383) -> (w379:T6)
      }
    }
  }
